vi "Queue - Manage - Polymorphic.vi"   [LabVIEW 2024, in "QMH Messaging.lvlib"]
uses:
  QMH Messaging.lvlib
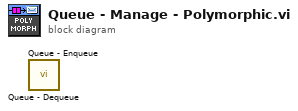
[diagram p0: block diagram]
diagram:
  n1 = call "Queue - Dequeue.vi"() -> ()  [unwired: 8 in, 4 out]
  n2 = call "Queue - Enqueue.vi"() -> ()  [unwired: 10 in, 2 out]
